vi "Write Config.vi"(8 "error in (no error)":errorcluster, 9 "Re-Init?":bool, 10 "ICM File In":path, 11 "All Channels in":refnum<class "All Channels Out.lvclass">) -> (0 "error out":errorcluster, 3 "All Channels out":refnum<class "All Channels Out.lvclass">)   [LabVIEW 2024, in "All Channels Out.lvclass"]
doc: "All Channels.lvclass:Write Config.vi\n\nThis VI writes the All Channels Class parameters to the ICM configuration file.\n\nInstrument Communication Module Version 1.0\nOctober, 2020 Original Code Consulting Davita Bird\n www.originalcode.com"
uses:
  All Channels Out.lvclass
  All Channels Out.lvclass/All Channels Out.ctl
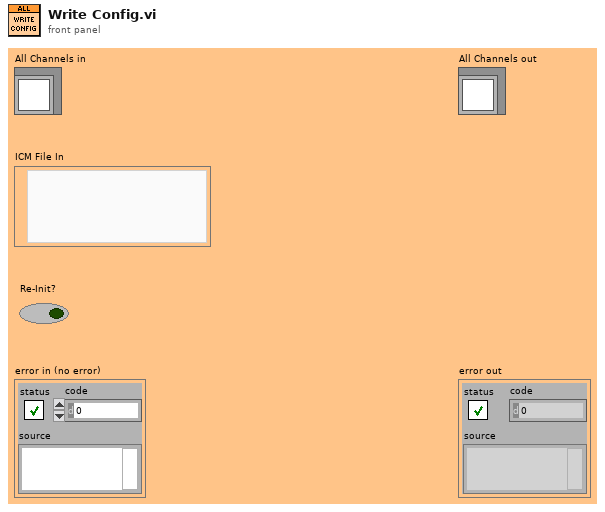
[diagram p1: front panel]
types:
  T1 = typedef "All Channels Type Def.ctl" = cluster{"Channel Names":string[], "Enabled":bool[], "Format Specifiers":string[], "String Header":string, "Use Same Format\nSpecifier \nFor All Channels":bool, "Delimiter":string, "Initial Value":dbl[], "Set Initial Values At Startup?":bool}
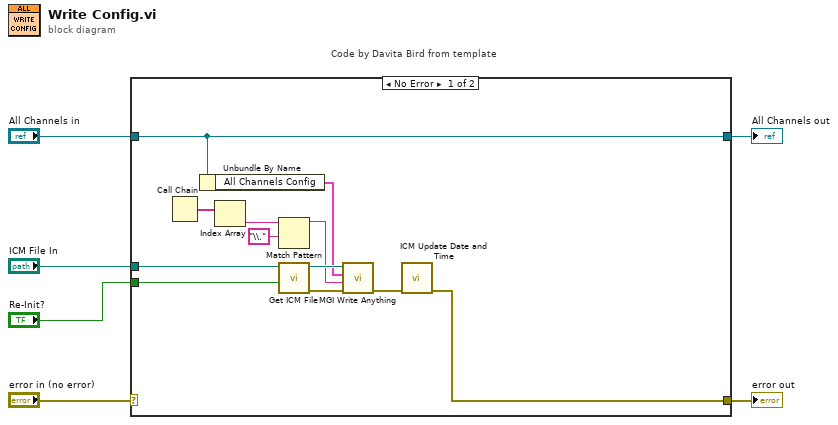
[diagram p0: block diagram]
diagram:
  n1 = case "Code by Davita Bird from template" shown="No Error" "error in (no error)" {
    selector: "error in (no error)" -> [_ w20]
    tunnel: [w7 w20] -> w5
    tunnel: [w15 w19] -> w3
    tunnel: "All Channels in" -> [w15 w19]
    tunnel: "ICM File In" -> [w10 _]
    tunnel: "Re-Init?" -> [w9 _]
    frame No Error {
      n2 = Call Chain() -> (call chain=w17:string[])
      n3 = Unbundle By Name(w15) -> ("All Channels Config"=w11:T1)
      n4 = Index Array(array=w17) -> (element=w16:string)  [unwired: 1 in]
      n5 = Match Pattern(string=w16, regular expression="\\.") -> (before substring=w12:string)  [unwired: 1 in, 3 out]
      n6 = call "Get ICM File.vi"("Re-Init?"=w9, "ICM File In"=w10) -> ("error out"=w14:errorcluster, "ICM File"=w13:path)  [unwired: 8 in]
      n7 = call "MGI Write Anything.vi"("Error In"=w14, "Section Name (Name of \"Anything\")"=w12, "Anything"=w11, "Path (dialog)"=w13) -> ("Error Out"=w8:errorcluster)  [unwired: 5 in, 2 out]
      n8 = call "ICM Update Date and Time.vi"("error in (no error)"=w8) -> ("error out"=w7:errorcluster)  [unwired: 9 in, 1 out]
    }
    frame Error {
    }
  }
  "error out" <- w5
  "All Channels out" <- w3
